vi "CU_Main_Function.vi"(8 "Stop Button Ref":refnum<vi>, 10 "Indicator Refs in":T4, 11 "Classifier Metaparameters in":T1={"Training Data Path"=path "", "Test Data Path"=path "", "True Labels Path"=path "", "SVM ClassifierOptions"={"Kernel"=enum."Linear", "Degree"=3, "Gamma"=1.0, "Coefficient"=0.0, "Sigma"=1.0, "Cache(MB)"=200.0}, "% of redundant features"=0.0, "Use equal number of trials?"=FALSE, "ClassifierQualityMeasure"=enum."Accuracy"} {"% of redundant features" min=0.0 max=100.0 step=1.0 scale=0.0..100.0}) -> (2 "Accuracies String out":string[](array[string]), 3 "Accuracies out":dbl[](array[numeric]) caption="Точность" format="%#_3g")   [LabVIEW 2016, in "Classifier.lvlib"]
uses:
  CU_metaIndicators.ctl
  CU_metaParameters.ctl
  <vilib>/vision/Classification.llb/IMAQ SVM Kernel Options.ctl
  CU_ClassifierQualityMeasure.ctl
  CU_ApplicationState.ctl
  ClassifierClass.lvclass
  ClassifierClass.lvclass/ClassifierClass.ctl
  CU_DataTypes.ctl
  CU_ClassifierTypes.ctl
  Classifier.lvlib
panel:
  out "Num of trials of each class":i32[](array[numeric]) caption="Число проб каждого класса"
  out "Num of Classes":i32 caption="Число классов"
  out "Number of Training Trials":i32 caption="Число обучающих проб"
  out "Number of Test Trials":i32 caption="Число тестовых проб"
  out "Number of Labels":i32 caption="Число меток классов"
  out "Iteration":i32 caption="Раунд кросс-проверки"
  out "Indices":i8[](array[numeric])
  # "This VI is a part of BCI Design library, http://www.ru-bci.org \nCopyright © 2020, Sotnikov Peter, All rights reserved. License: GNU GPLv3"
  # "Метод опорных векторов"
  # "Метод k ближайших соседей"
  # "Многослойный персептрон"
  # "Результаты чтения данных"
  # "Комитет классификаторов на основе метода опорных векторов"
  # "Классификатор на основе расстояния Махалонобиса"
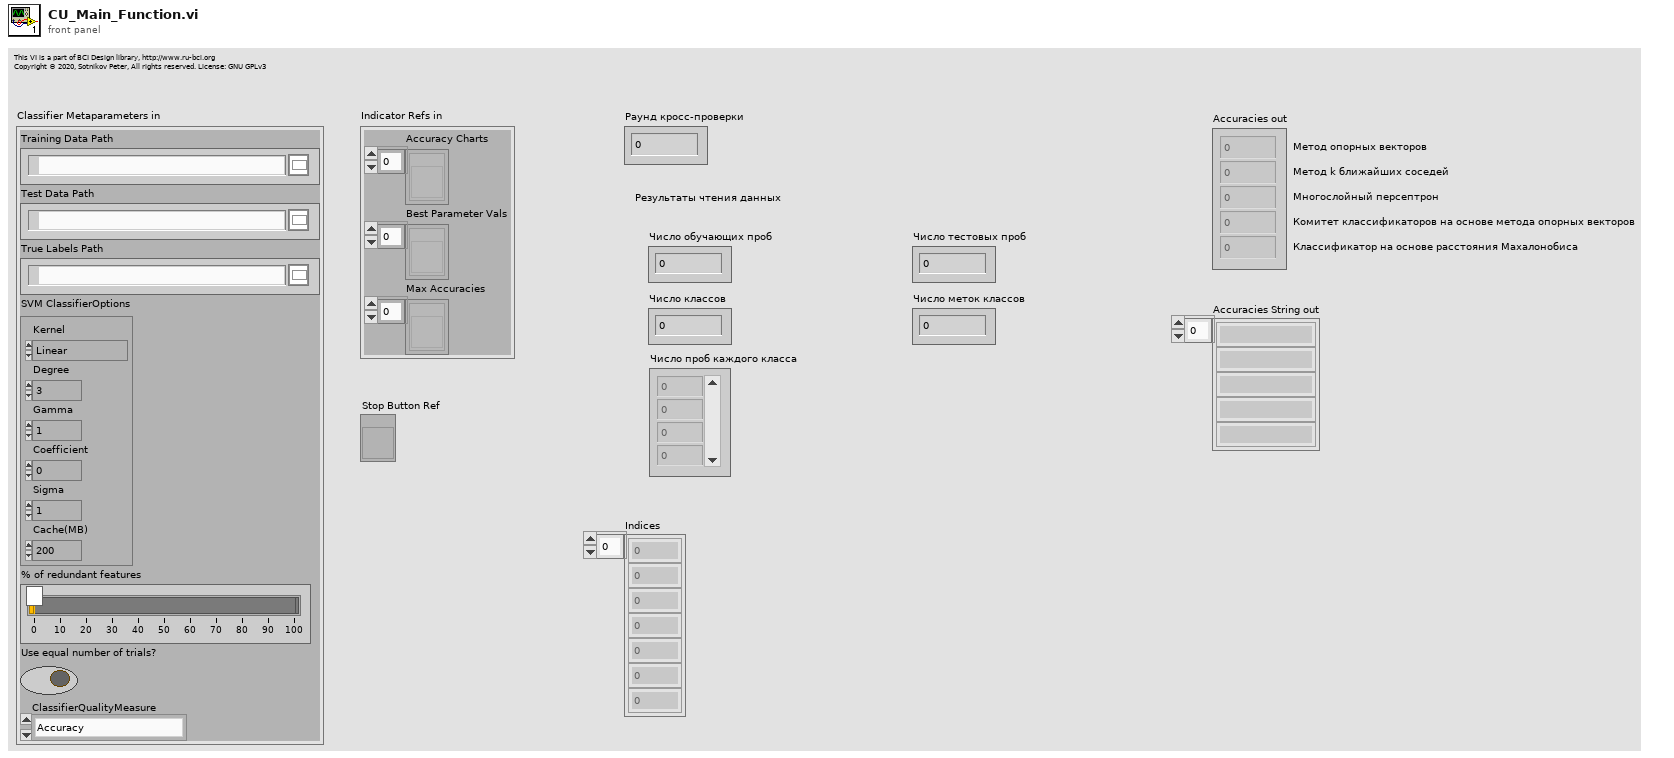
[diagram p1: front panel]
types:
  T1 = typedef "Classifier.lvlib/CU_metaParameters.ctl" = cluster{"Training Data Path":path, "Test Data Path":path, "True Labels Path":path, "SVM ClassifierOptions":T2, "% of redundant features":dbl, "Use equal number of trials?":bool, "ClassifierQualityMeasure":T3}
  T2 = typedef "IMAQ SVM Kernel Options.ctl" = cluster{"Kernel":enum32{"Linear", "Polynomial", "Gaussian", "RBF"}, "Degree":i32, "Gamma":dbl, "Coefficient":dbl, "Sigma":dbl, "Cache(MB)":dbl}
  T3 = typedef "Classifier.lvlib/CU_ClassifierQualityMeasure.ctl" = enum16{"Accuracy", "Cohen's kappa"}
  T4 = typedef "Classifier.lvlib/CU_metaIndicators.ctl" = cluster{"Accuracy Charts":refnum<vi>[], "Best Parameter Vals":refnum<vi>[], "Max Accuracies":refnum<vi>[]}
  T5 = typedef "Classifier.lvlib/CU_ApplicationState.ctl" = enum16{"Initialiaze", "Work", "On test data", "Stop", "InitCrossValidation", "CrossValidation"}
  T6 = typedef "Classifier.lvlib/CU_DataTypes.ctl" = enum16{"Training Data", "Test Data", "Training Data (cross-check)", "Test Data (cross-check)"}
  T7 = typedef "Classifier.lvlib/CU_ClassifierTypes.ctl" = enum16{"Multilayer perceptron", "k NN Classifier", "SVM Committee", "Mahalanobis distance", "SVM Classifier"}
  T8 = cluster{"Training Data Path":path, "Test Data Path":path, "True Labels Path":path}
  T9 = cluster{"Number of Classes":i32, "NumberOfTrials":i32, "NumberOfTrials":i32, "Number of labels":i32}
  T10 = typedef "IMAQ Classifier Session.ctl" = refnum<k1>
  T11 = typedef "NILabs_MLT.lvlib/ml_BP_Project.ctl" = cluster{"Training Data":T12, "Normalize Info":T13, "3-layer NN":T14, "Ternimal Condition":T15}
  T12 = typedef "NILabs_MLT.lvlib/ml_BP_Data.ctl" = cluster{"dim in":i32, "dim out":i32, "# samples":i32, "Input":dbl[][], "Output":dbl[][]}
  T13 = typedef "NILabs_MLT.lvlib/ml_BP_Normalize Data.ctl" = cluster{"input min":dbl[], "input max":dbl[], "output min":dbl[], "output max":dbl[]}
  T14 = typedef "NILabs_MLT.lvlib/ml_BP_3layer Feedforward.ctl" = cluster{"# input neuron ":i32, "# hidden neuron":i32, "# output neuron":i32, "Weight (I->H)":dbl[][], "Weight (H->O)":dbl[][], "Output":dbl[][], "Hidden Out":dbl[][], "Derivation Output":dbl[][], "Derivation Hidden":dbl[][], "dw (I->H)":dbl[][], "dw (H->O)":dbl[][]}
  T15 = typedef "NILabs_MLT.lvlib/ml_BP_Terminal Condition.ctl" = cluster{"min MSE":dbl, "min delta MSE":dbl, "min step length":dbl, "max iteration":dbl}
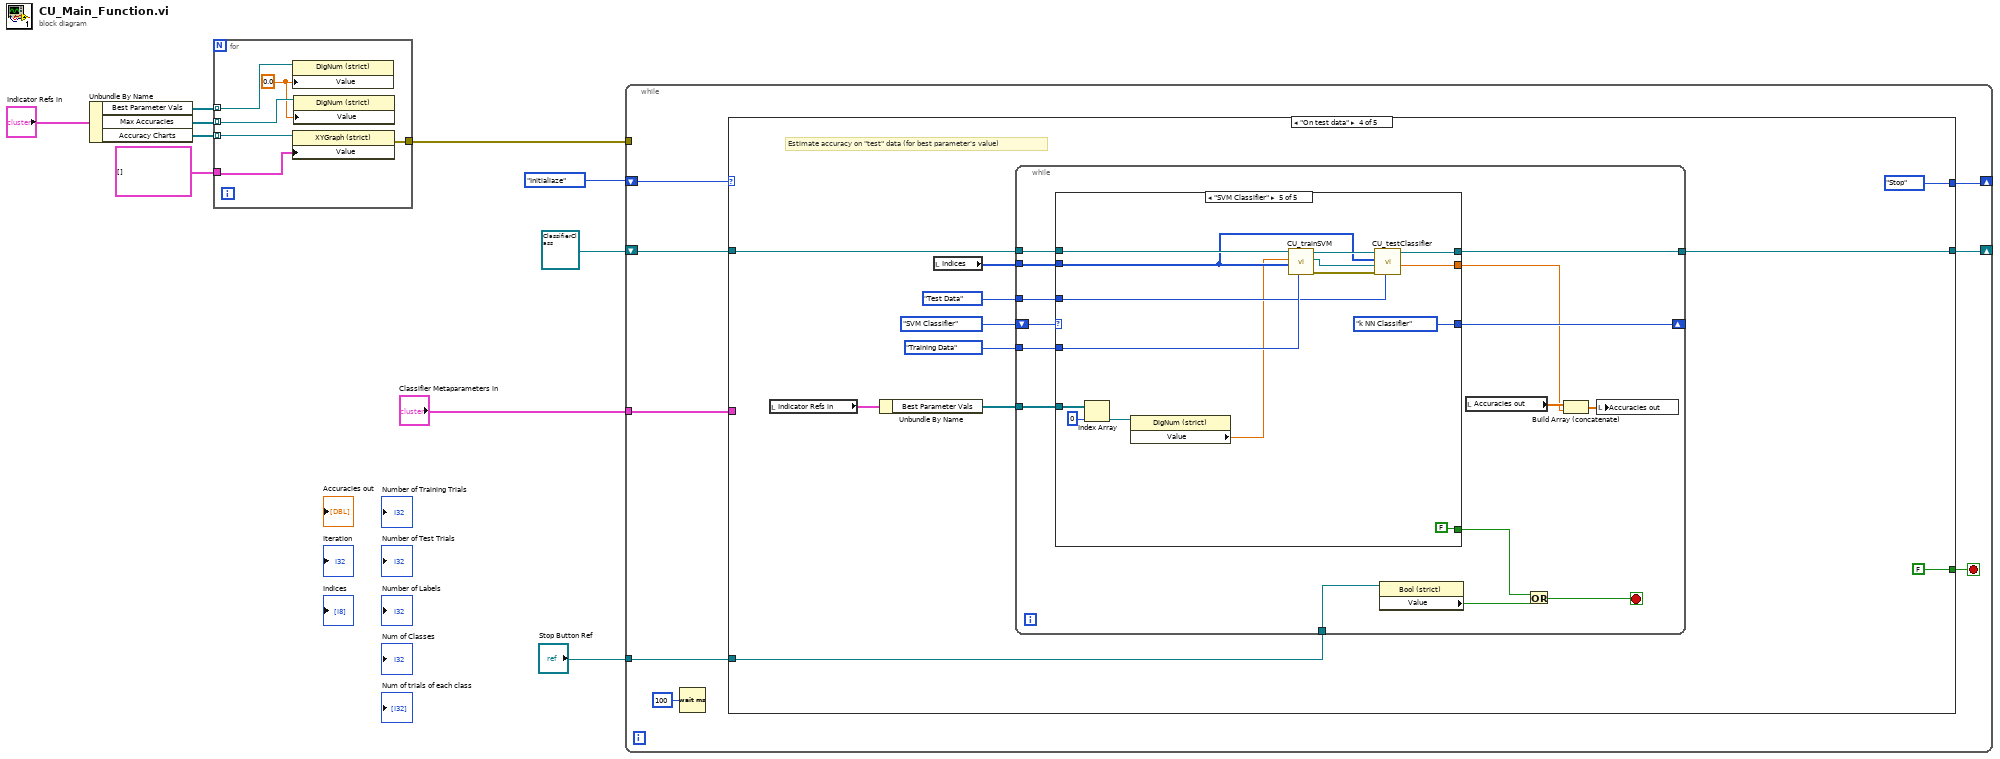
[diagram p0: block diagram]
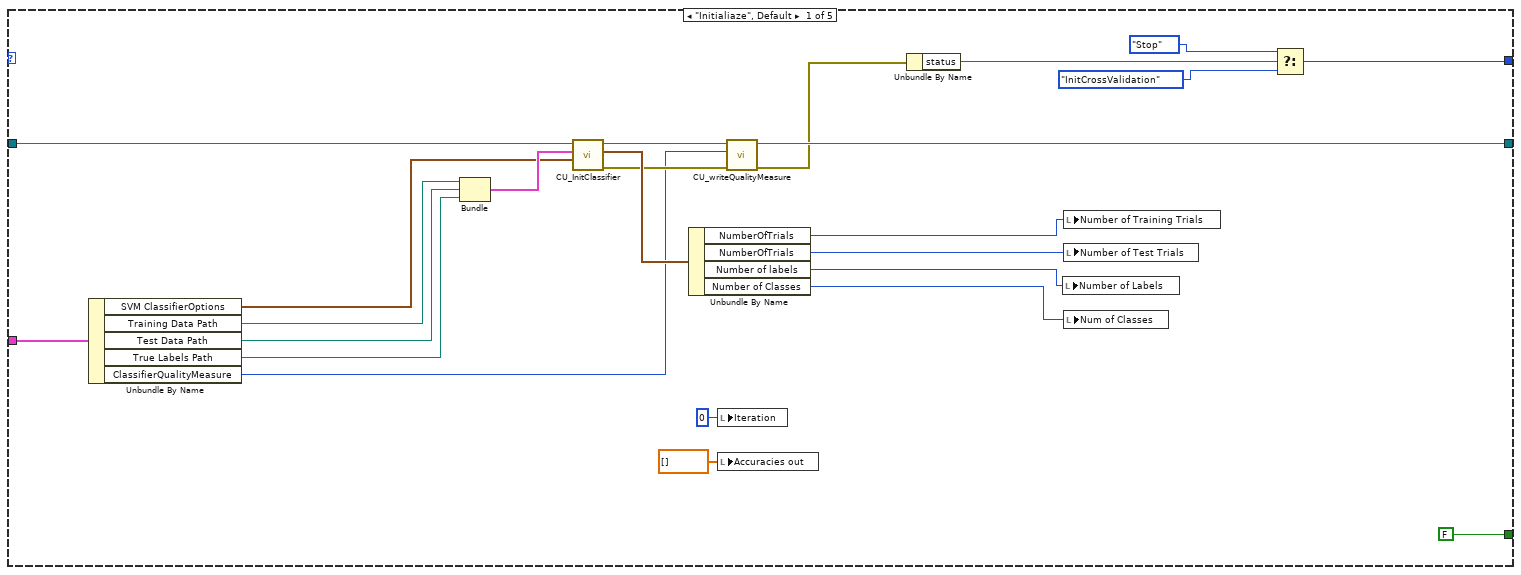
[diagram p2: hidden frame]
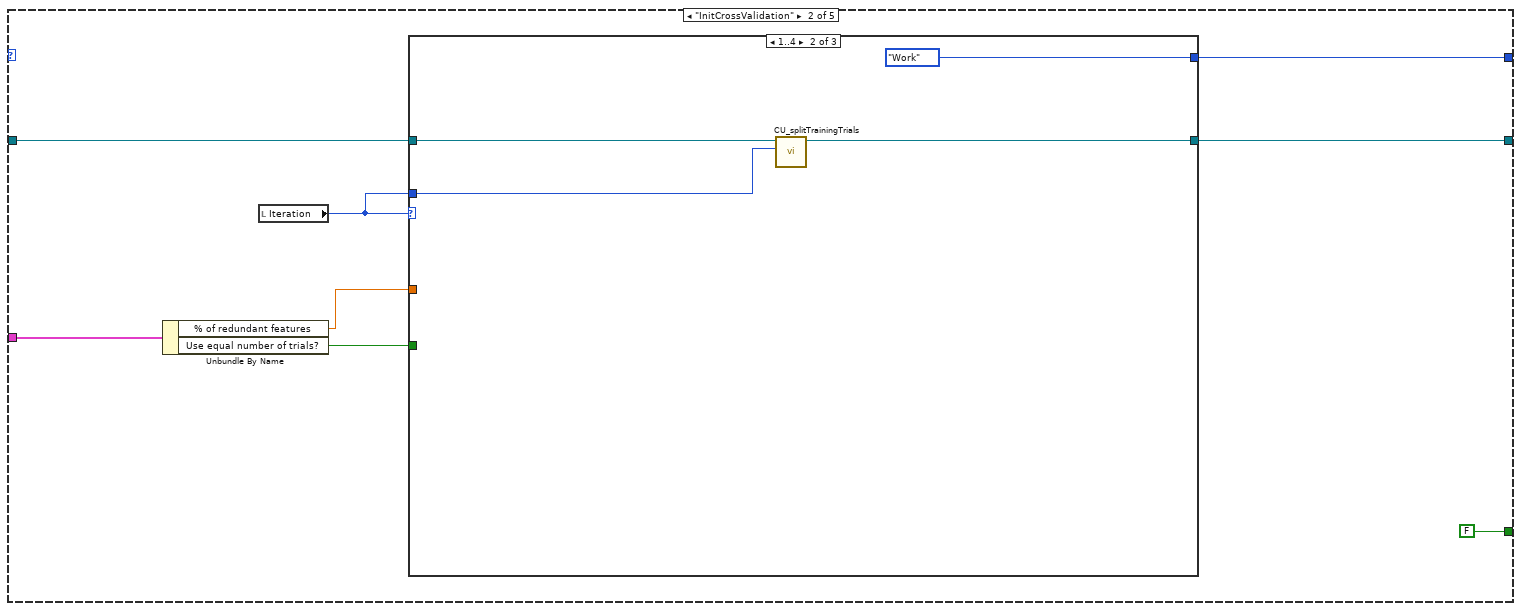
[diagram p3: hidden frame]
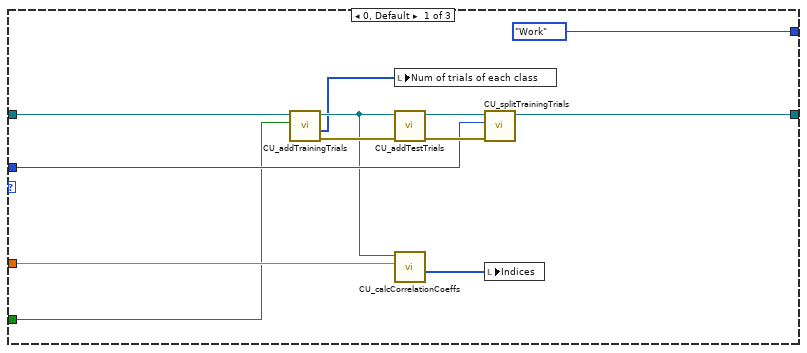
[diagram p4: hidden frame]
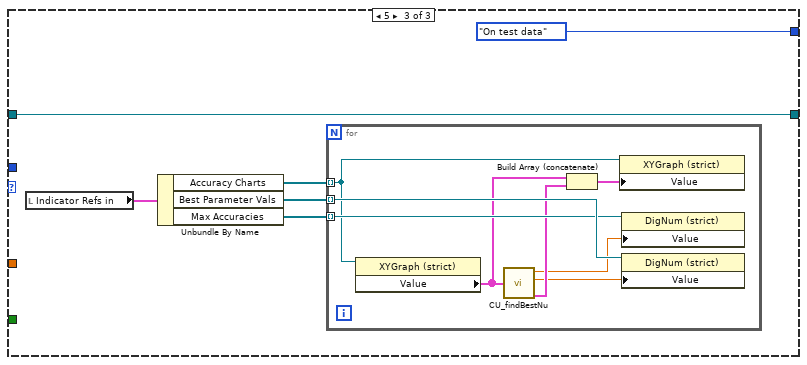
[diagram p5: hidden frame]
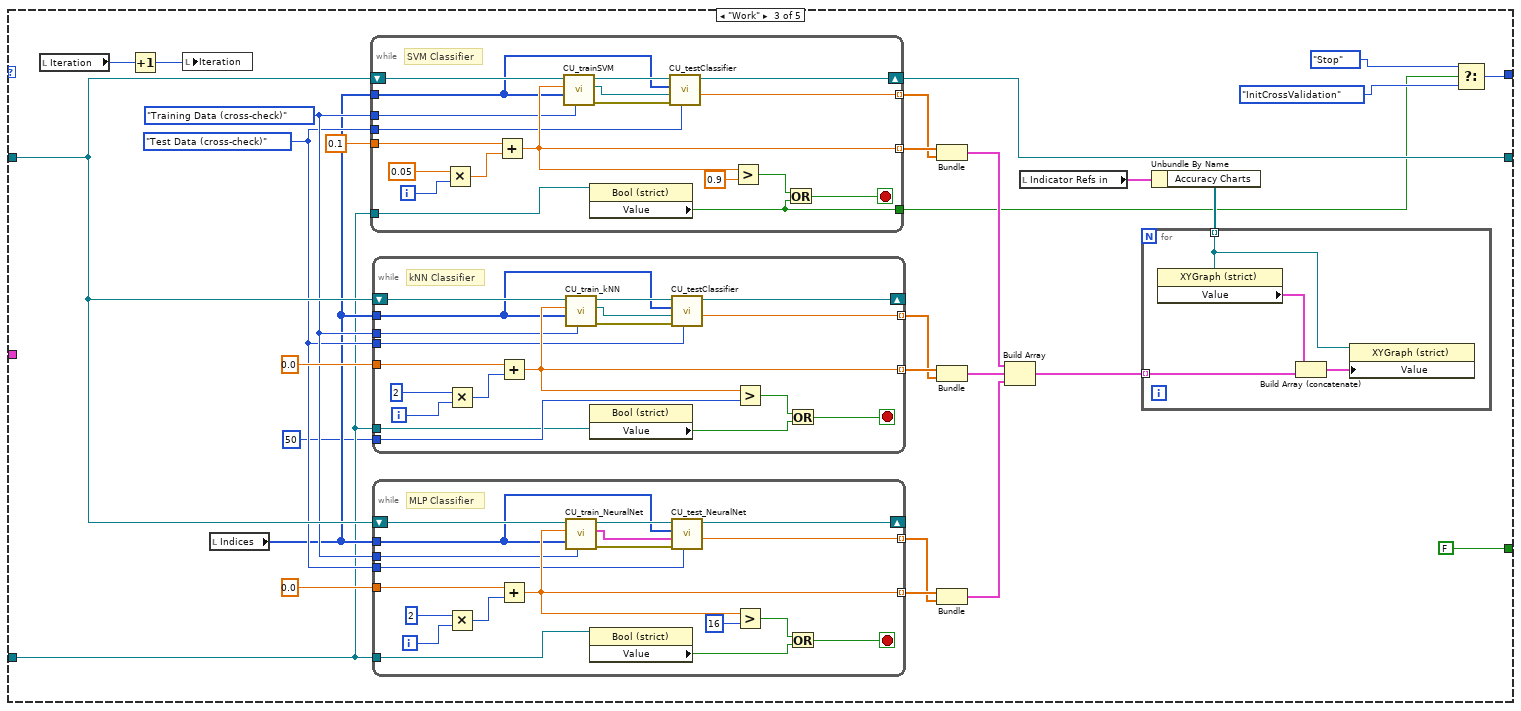
[diagram p6: hidden frame]
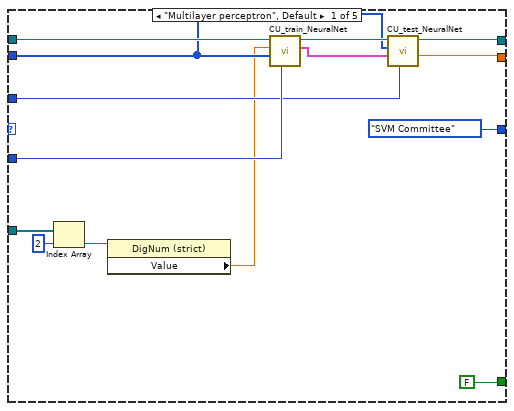
[diagram p7: hidden frame]
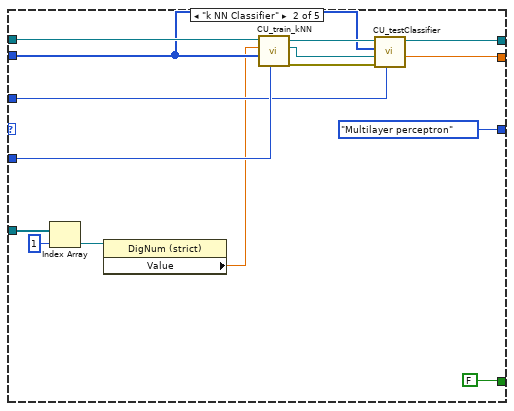
[diagram p8: hidden frame]
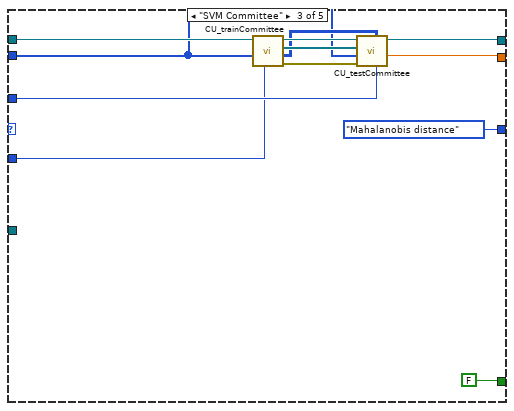
[diagram p9: hidden frame]
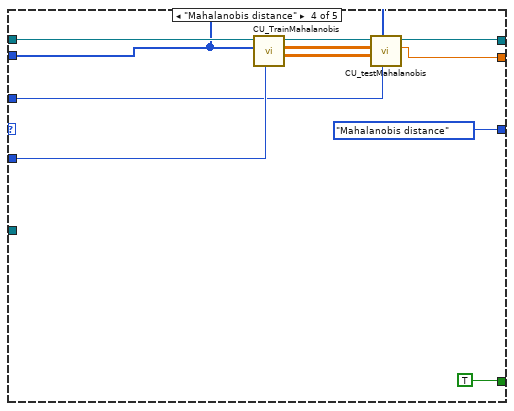
[diagram p10: hidden frame]
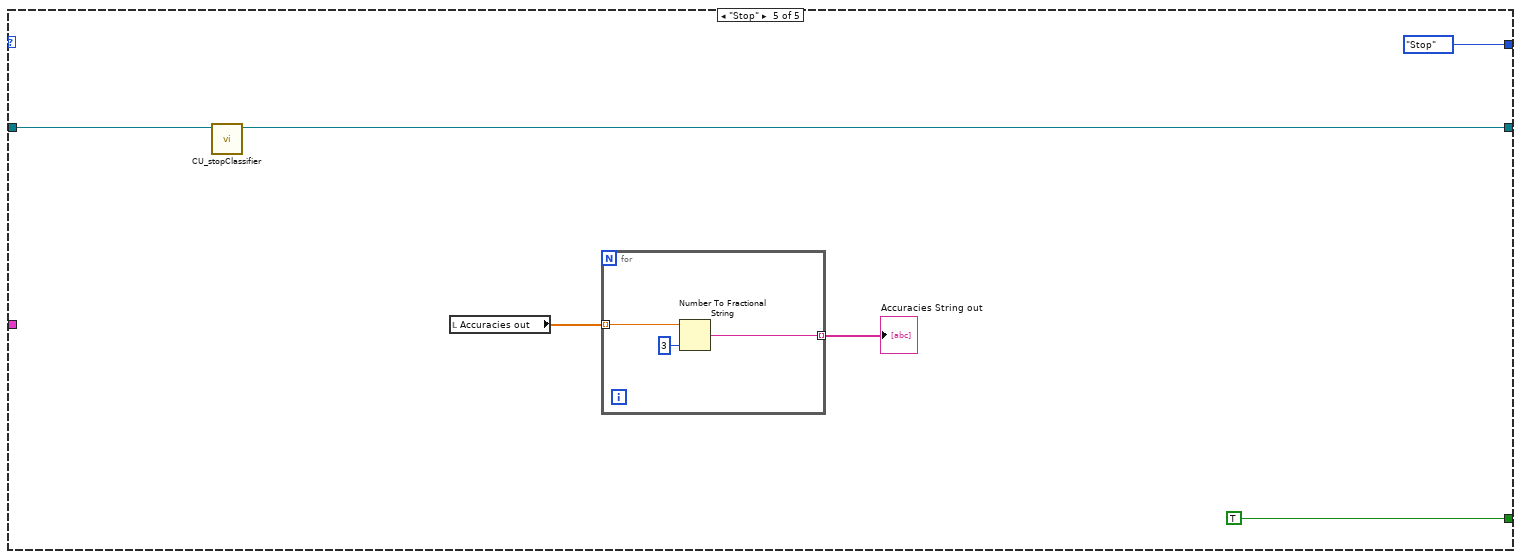
[diagram p11: hidden frame]
diagram:
  n1 = Unbundle By Name("Indicator Refs in") -> ("Best Parameter Vals"=w4:refnum<vi>[], "Max Accuracies"=w3:refnum<vi>[], "Accuracy Charts"=w7:refnum<vi>[])
  n2 = for {
    tunnel: w7 -> [w16] mode=indexing
    tunnel: [w15] -> w6
    tunnel: w4 -> [w14] mode=indexing
    tunnel: w3 -> [w13] mode=indexing
    tunnel: cluster{dbl[], dbl[]}[] [] ("Value") -> [w11]
    w12 = 0.0 ("Value")
    n3 = property class="XYGraph (strict)"(reference=w16, "Value"=w11) -> (error out=w15:errorcluster)  [unwired: 1 in, 1 out]
    n4 = property class="DigNum (strict)"(reference=w14, "Value"=w12) -> ()  [unwired: 1 in, 2 out]
    n5 = property class="DigNum (strict)"(reference=w13, "Value"=w12) -> ()  [unwired: 1 in, 2 out]
  }
  n6 = while {
    shift-right: [w23] -> _
    shift-left: CU_ApplicationState."Initialiaze" ("Application State") -> [w24]
    shift-right: [w19] -> _
    shift-left: refnum<class "ClassifierClass.lvclass"> refnum ("ClassifierClass.lvclass") -> [w20]
    tunnel: w6 -> [_]
    tunnel: "Stop Button Ref" -> [w18]
    tunnel: "Classifier Metaparameters in" -> [w17]
    stop <- w22 stop-if-true
    n7 = Wait (ms)(milliseconds to wait=u32 100) -> ()  [unwired: 1 out]
    n8 = case shown="\"On test data\"" w24 {
      tunnel: [w48 w55 w89 CU_ApplicationState."Stop" ("f") CU_ApplicationState."Stop" ("f")] -> w23
      tunnel: [FALSE FALSE FALSE FALSE TRUE] -> w22
      tunnel: w20 -> [w46 w56 w107 w183 w273]
      tunnel: [w26 w53 w113 w184 w272] -> w19
      tunnel: w18 -> [_ _ w92 w177 _]
      tunnel: w17 -> [w36 w51 _ _ _]
      frame "Initialiaze", Default {
        n9 = Unbundle By Name(w36) -> ("SVM ClassifierOptions"=w32:T2, "Training Data Path"=w35:path, "Test Data Path"=w34:path, "True Labels Path"=w33:path, "ClassifierQualityMeasure"=w27:T3)
        n10 = Bundle("Training Data Path"=w35, "Test Data Path"=w34, "True Labels Path"=w33) -> (w43:T8)  [unwired: 1 in]
        n11 = call "CU_InitClassifier.vi"("Kernel Options"=w32, "Paths"=w43, "ClassifierClass in"=w46) -> ("error out"=w28:errorcluster, "Number of Trials"=w41:T9, "ClassifierClass out"=w29:refnum<class "ClassifierClass.lvclass">)  [unwired: 6 in]
        n12 = Unbundle By Name(w41) -> ("NumberOfTrials"=w40:i32, "NumberOfTrials"=w39:i32, "Number of labels"=w38:i32, "Number of Classes"=w37:i32)
        n13 = local write "Iteration"(0 ("Iteration")) -> ()
        n14 = local write "Accuracies out"(dbl[] [] ("Accuracies out")) -> ()
        n15 = call "CU_writeQualityMeasure.vi"("error in (no error)"=w28, "ClassifierQualityMeasure in"=w27, "ClassifierClass in"=w29) -> ("error out"=w25:errorcluster, "ClassifierClass out"=w26:refnum<class "ClassifierClass.lvclass">)  [unwired: 7 in]
        n16 = Unbundle By Name(w25) -> ("status"=w42:bool)
        n17 = local write "Number of Labels"(w38) -> ()
        n18 = local write "Number of Training Trials"(w40) -> ()
        n19 = local write "Number of Test Trials"(w39) -> ()
        n20 = local write "Num of Classes"(w37) -> ()
        n21 = Select(t=CU_ApplicationState."Stop" ("Application State"), s=w42, f=CU_ApplicationState."InitCrossValidation") -> (s? t:f=w48:T5)
      }
      frame "InitCrossValidation" {
        n22 = Unbundle By Name(w51) -> ("% of redundant features"=w50:dbl, "Use equal number of trials?"=w49:bool)
        n23 = local read "Iteration"() -> (w52:i32)
        n24 = case shown="1..4" w52 {
          tunnel: w56 -> [w68 w72 w78]
          tunnel: [w65 w71 w78] -> w53
          tunnel: w52 -> [w63 w70 _]
          tunnel: [CU_ApplicationState."Work" ("Application State") CU_ApplicationState."Work" ("Application State") CU_ApplicationState."On test data" ("Application State")] -> w55
          tunnel: w50 -> [w59 _ _]
          tunnel: w49 -> [w58 _ _]
          frame 0, Default {
            n25 = call "CU_addTrainingTrials.vi"("Use equal number of trials?"=w58, "ClassifierClass in"=w68) -> ("error out"=w67:errorcluster, "Num of Trials of each Class"=w57:i32[], "ClassifierClass out"=w61:refnum<class "ClassifierClass.lvclass">)  [unwired: 6 in, 1 out]
            n26 = local write "Num of trials of each class"(w57) -> ()
            n27 = call "CU_addTestTrials.vi"("error in (no error)"=w67, "ClassifierClass in"=w61) -> ("error out"=w64:errorcluster, "ClassifierClass out"=w66:refnum<class "ClassifierClass.lvclass">)  [unwired: 6 in, 2 out]
            n28 = call "CU_calcCorrelationCoeffs.vi"("Percent in"=w59, "ClassifierClass in"=w61) -> ("Indicies"=w60:i16[])  [unwired: 6 in, 3 out]
            n29 = call "CU_splitTrainingTrials.vi"("error in (no error)"=w64, "Iteration"=w63, "ClassifierClass in"=w66) -> ("ClassifierClass out"=w65:refnum<class "ClassifierClass.lvclass">)  [unwired: 5 in, 3 out]
            n30 = local write "Indices"(w60) -> ()
          }
          frame 1..4 {
            n31 = call "CU_splitTrainingTrials.vi"("Iteration"=w70, "ClassifierClass in"=w72) -> ("ClassifierClass out"=w71:refnum<class "ClassifierClass.lvclass">)  [unwired: 6 in, 3 out]
          }
          frame 5 {
            n32 = local read "Indicator Refs in"() -> (w76:T4)
            n33 = Unbundle By Name(w76) -> ("Accuracy Charts"=w75:refnum<vi>[], "Best Parameter Vals"=w74:refnum<vi>[], "Max Accuracies"=w73:refnum<vi>[])
            n34 = for {
              tunnel: w75 -> [w84] mode=indexing
              tunnel: w74 -> [w86] mode=indexing
              tunnel: w73 -> [w85] mode=indexing
              n35 = property class="XYGraph (strict)"(reference=w84) -> ("Value"=w82:cluster{dbl[], dbl[]}[])  [unwired: 1 in, 2 out]
              n36 = call "CU_findBestNu.vi"("Accuracy Graph"=w82) -> ("Max Average Accuracy"=w80:dbl, "Best Value"=w79:dbl, "Average Accuracy"=w83:cluster{dbl[], dbl[]})  [unwired: 7 in]
              n37 = Build Array (concatenate)(w82, w83) -> (w81:cluster{dbl[], dbl[]}[])
              n38 = property class="XYGraph (strict)"(reference=w84, "Value"=w81) -> ()  [unwired: 1 in, 2 out]
              n39 = property class="DigNum (strict)"(reference=w85, "Value"=w80) -> ()  [unwired: 1 in, 2 out]
              n40 = property class="DigNum (strict)"(reference=w86, "Value"=w79) -> ()  [unwired: 1 in, 2 out]
            }
          }
        }
      }
      frame "Work" {
        w101 = CU_DataTypes."Test Data (cross-check)" ("DataTypes")
        w102 = CU_DataTypes."Training Data (cross-check)" ("DataTypes")
        n41 = local read "Iteration"() -> (w110:i32)
        n42 = Increment(x=w110) -> (x+1=w109:i32)
        n43 = local write "Iteration"(w109) -> ()
        n44 = local read "Indices"() -> (w100:i8[])
        n45 = while {
          tunnel: 0.1 -> [w172]
          tunnel: [w170] -> w111 mode=indexing
          shift-right: [w169] -> w113
          shift-left: w107 -> [w176]
          tunnel: [w163] -> w112 mode=indexing
          tunnel: w102 -> [w162]
          tunnel: w101 -> [w161]
          tunnel: w100 -> [w160]
          tunnel: w92 -> [w159]
          tunnel: [w158] -> w88
          i -> [w175]
          stop <- w166 stop-if-true
          # "SVM Classifier"
          n46 = Multiply(x=0.05, y=w175) -> (x*y=w173:dbl)
          n47 = Add(x=w172, y=w173) -> (x+y=w163:dbl)
          n48 = call "CU_trainSVM.vi"("Train Data"=w162, "Indices"=w160, "Nu Value"=w163, "ClassifierClass in"=w176) -> ("error out"=w165:errorcluster, "Classifier Session out"=w164:T10, "ClassifierClass out"=w171:refnum<class "ClassifierClass.lvclass">)  [unwired: 5 in]
          n49 = property class="Bool (strict)"(reference=w159) -> ("Value"=w158:bool)  [unwired: 1 in, 2 out]
          n50 = call "CU_testClassifier.vi"("DataTypes"=w161, "error in"=w165, "Classifier Session Ref"=w164, "Indices"=w160, "ClassifierClass in"=w171) -> ("Accuracy"=w170:dbl, "ClassifierClass out"=w169:refnum<class "ClassifierClass.lvclass">)  [unwired: 3 in, 2 out]
          n51 = Greater?(x=w163, y=0.9) -> (0:w167:bool)
          n52 = Or(x=w167, y=w158) -> (x .or. y?=w166:bool)
        }
        n53 = while {
          tunnel: 0.0 -> [w153]
          tunnel: [w151] -> w105 mode=indexing
          shift-right: [w150] -> _
          shift-left: w107 -> [w157]
          tunnel: 50 -> [w145]
          tunnel: [w144] -> w106 mode=indexing
          tunnel: w102 -> [w143]
          tunnel: w101 -> [w142]
          tunnel: w100 -> [w141]
          tunnel: w92 -> [w139]
          i -> [w156]
          stop <- w148 stop-if-true
          # "kNN Classifier"
          n54 = Multiply(x=2, y=w156) -> (x*y=w154:i32)
          n55 = Add(x=w153, y=w154) -> (x+y=w144:dbl)
          n56 = call "CU_train_kNN.vi"("DataTypes"=w143, "Indices"=w141, "k value"=w144, "ClassifierClass in"=w157) -> ("error out"=w147:errorcluster, "Classifier Session out"=w146:T10, "ClassifierClass out"=w152:refnum<class "ClassifierClass.lvclass">)  [unwired: 5 in]
          n57 = property class="Bool (strict)"(reference=w139) -> ("Value"=w140:bool)  [unwired: 1 in, 2 out]
          n58 = call "CU_testClassifier.vi"("DataTypes"=w142, "error in"=w147, "Classifier Session Ref"=w146, "Indices"=w141, "ClassifierClass in"=w152) -> ("Accuracy"=w151:dbl, "ClassifierClass out"=w150:refnum<class "ClassifierClass.lvclass">)  [unwired: 3 in, 2 out]
          n59 = Greater?(x=w144, y=w145) -> (0:w149:bool)
          n60 = Or(x=w149, y=w140) -> (x .or. y?=w148:bool)
        }
        n61 = while {
          tunnel: [w134] -> w93 mode=indexing
          shift-right: [w133] -> _
          shift-left: w107 -> [w138]
          tunnel: [w128] -> w103 mode=indexing
          tunnel: 0.0 -> [w127]
          tunnel: w102 -> [w124]
          tunnel: w101 -> [w123]
          tunnel: w100 -> [w122]
          tunnel: w92 -> [w121]
          i -> [w137]
          stop <- w131 stop-if-true
          # "MLP Classifier"
          n62 = Multiply(x=2, y=w137) -> (x*y=w136:i32)
          n63 = Add(x=w127, y=w136) -> (x+y=w128:dbl)
          n64 = call "CU_train_NeuralNet.vi"("DataTypes"=w124, "Indices"=w122, "# of hidden neuron"=w128, "ClassifierClass in"=w138) -> ("error out"=w130:errorcluster, "ANN out"=w129:T11, "ClassifierClass out"=w135:refnum<class "ClassifierClass.lvclass">)  [unwired: 4 in, 1 out]
          n65 = property class="Bool (strict)"(reference=w121) -> ("Value"=w120:bool)  [unwired: 1 in, 2 out]
          n66 = call "CU_test_NeuralNet.vi"("DataTypes"=w123, "error in"=w130, "ANN in"=w129, "Indices"=w122, "ClassifierClass in"=w135) -> ("Accuracy"=w134:dbl, "ClassifierClass out"=w133:refnum<class "ClassifierClass.lvclass">)  [unwired: 3 in, 2 out]
          n67 = Greater?(x=w128, y=16) -> (0:w132:bool)
          n68 = Or(x=w132, y=w120) -> (x .or. y?=w131:bool)
        }
        n69 = Bundle(w112, w111) -> (w97:cluster{dbl[], dbl[]})  [unwired: 1 in]
        n70 = Bundle(w106, w105) -> (w98:cluster{dbl[], dbl[]})  [unwired: 1 in]
        n71 = Bundle(w103, w93) -> (w96:cluster{dbl[], dbl[]})  [unwired: 1 in]
        n72 = Build Array(w97, w98, w96) -> (w94:cluster{dbl[], dbl[]}[])
        n73 = local read "Indicator Refs in"() -> (w99:T4)
        n74 = Unbundle By Name(w99) -> ("Accuracy Charts"=w95:refnum<vi>[])
        n75 = for {
          tunnel: w95 -> [w119] mode=indexing
          tunnel: w94 -> [w117] mode=indexing
          n76 = property class="XYGraph (strict)"(reference=w119) -> ("Value"=w118:cluster{dbl[], dbl[]}[])  [unwired: 1 in, 2 out]
          n77 = Build Array (concatenate)(w118, w117) -> (w116:cluster{dbl[], dbl[]}[])
          n78 = property class="XYGraph (strict)"(reference=w119, "Value"=w116) -> ()  [unwired: 1 in, 2 out]
        }
        n79 = Select(t=CU_ApplicationState."Stop" ("Application State"), s=w88, f=CU_ApplicationState."InitCrossValidation") -> (s? t:f=w89:T5)
      }
      frame "On test data" {
        # "Estimate accuracy on \"test\" data (for best parameter's value)"
        n80 = local read "Indicator Refs in"() -> (w179:T4)
        n81 = Unbundle By Name(w179) -> ("Best Parameter Vals"=w178:refnum<vi>[])
        n82 = local read "Indices"() -> (w180:i8[])
        n83 = while {
          shift-right: [w201] -> _
          shift-left: CU_ClassifierTypes."SVM Classifier" ("ClassifierTypes") -> [w202]
          tunnel: w183 -> [w200]
          tunnel: [w199] -> w184
          tunnel: CU_DataTypes."Training Data" ("Train Data") -> [w198]
          tunnel: CU_DataTypes."Test Data" ("DataTypes") -> [w197]
          tunnel: w180 -> [w193]
          tunnel: w178 -> [w192]
          tunnel: w177 -> [w191]
          stop <- w188 stop-if-true
          n84 = case shown="\"SVM Classifier\"" w202 {
            tunnel: [FALSE FALSE FALSE TRUE FALSE] -> w189
            tunnel: [CU_ClassifierTypes."SVM Committee" ("ClassifierTypes") CU_ClassifierTypes."Multilayer perceptron" ("ClassifierTypes") CU_ClassifierTypes."Mahalanobis distance" ("ClassifierTypes") CU_ClassifierTypes."Mahalanobis distance" ("ClassifierTypes") CU_ClassifierTypes."k NN Classifier" ("ClassifierTypes")] -> w201
            tunnel: w200 -> [w214 w225 w238 w251 w266]
            tunnel: [w212 w226 w237 w250 w265] -> w199
            tunnel: w198 -> [w209 w223 w234 w247 w263]
            tunnel: w197 -> [w208 w222 w235 w246 w262]
            tunnel: [w210 w224 w233 w245 w261] -> w194
            tunnel: w193 -> [w207 w221 w232 w244 w260]
            tunnel: w192 -> [w206 w220 _ _ w258]
            frame "Multilayer perceptron", Default {
              n85 = Index Array(array=w206, index=2) -> (element=w204:refnum<vi>)
              n86 = property class="DigNum (strict)"(reference=w204) -> ("Value"=w203:dbl)  [unwired: 1 in, 2 out]
              n87 = call "CU_train_NeuralNet.vi"("DataTypes"=w209, "Indices"=w207, "# of hidden neuron"=w203, "ClassifierClass in"=w214) -> ("ANN out"=w211:T11, "ClassifierClass out"=w213:refnum<class "ClassifierClass.lvclass">)  [unwired: 4 in, 2 out]
              n88 = call "CU_test_NeuralNet.vi"("DataTypes"=w208, "ANN in"=w211, "Indices"=w207, "ClassifierClass in"=w213) -> ("Accuracy"=w210:dbl, "ClassifierClass out"=w212:refnum<class "ClassifierClass.lvclass">)  [unwired: 4 in, 2 out]
            }
            frame "k NN Classifier" {
              n89 = Index Array(array=w220, index=1) -> (element=w218:refnum<vi>)
              n90 = property class="DigNum (strict)"(reference=w218) -> ("Value"=w217:dbl)  [unwired: 1 in, 2 out]
              n91 = call "CU_train_kNN.vi"("DataTypes"=w223, "Indices"=w221, "k value"=w217, "ClassifierClass in"=w225) -> ("error out"=w228:errorcluster, "Classifier Session out"=w229:T10, "ClassifierClass out"=w227:refnum<class "ClassifierClass.lvclass">)  [unwired: 5 in]
              n92 = call "CU_testClassifier.vi"("DataTypes"=w222, "error in"=w228, "Classifier Session Ref"=w229, "Indices"=w221, "ClassifierClass in"=w227) -> ("Accuracy"=w224:dbl, "ClassifierClass out"=w226:refnum<class "ClassifierClass.lvclass">)  [unwired: 3 in, 2 out]
            }
            frame "SVM Committee" {
              n93 = call "CU_trainCommittee.vi"("DataTypes"=w234, "Indices"=w232, "ClassifierClass in"=w238) -> ("error out"=w240:errorcluster, "Classification Distribution"=w236:i32[][][], "Classifier Refs out"=w241:T10[], "ClassifierClass out"=w239:refnum<class "ClassifierClass.lvclass">)  [unwired: 5 in]
              n94 = call "CU_testCommittee.vi"("ClassifierClass in"=w239, "Classifier Refs in"=w241, "Indices"=w232, "error in"=w240, "Classification Distribution"=w236, "DataTypes"=w235) -> ("ClassifierClass out"=w237:refnum<class "ClassifierClass.lvclass">, "Accuracy"=w233:dbl)  [unwired: 2 out]
            }
            frame "Mahalanobis distance" {
              n95 = call "CU_TrainMahalanobis.vi"("DataTypes"=w247, "Indices"=w244, "ClassifierClass in"=w251) -> ("Mean vectors"=w252:dbl[][], "Covariance matricies"=w253:dbl[][][], "ClassifierClass out"=w254:refnum<class "ClassifierClass.lvclass">)  [unwired: 5 in, 1 out]
              n96 = call "CU_testMahalanobis.vi"("DataTypes"=w246, "Indices"=w244, "Mean vectors"=w252, "Covariance matricies"=w253, "ClassifierClass in"=w254) -> ("Accuracy"=w245:dbl, "ClassifierClass out"=w250:refnum<class "ClassifierClass.lvclass">)  [unwired: 3 in, 2 out]
            }
            frame "SVM Classifier" {
              n97 = Index Array(array=w258, index=0) -> (element=w256:refnum<vi>)
              n98 = property class="DigNum (strict)"(reference=w256) -> ("Value"=w255:dbl)  [unwired: 1 in, 2 out]
              n99 = call "CU_trainSVM.vi"("Train Data"=w263, "Indices"=w260, "Nu Value"=w255, "ClassifierClass in"=w266) -> ("error out"=w268:errorcluster, "Classifier Session out"=w269:T10, "ClassifierClass out"=w267:refnum<class "ClassifierClass.lvclass">)  [unwired: 5 in]
              n100 = call "CU_testClassifier.vi"("DataTypes"=w262, "error in"=w268, "Classifier Session Ref"=w269, "Indices"=w260, "ClassifierClass in"=w267) -> ("Accuracy"=w261:dbl, "ClassifierClass out"=w265:refnum<class "ClassifierClass.lvclass">)  [unwired: 3 in, 2 out]
            }
          }
          n101 = property class="Bool (strict)"(reference=w191) -> ("Value"=w190:bool)  [unwired: 1 in, 2 out]
          n102 = local read "Accuracies out"() -> (w196:dbl[])
          n103 = Or(x=w189, y=w190) -> (x .or. y?=w188:bool)
          n104 = Build Array (concatenate)(w196, w194) -> (w195:dbl[])
          n105 = local write "Accuracies out"(w195) -> ()
        }
      }
      frame "Stop" {
        n106 = call "CU_stopClassifier.vi"("ClassifierClass in"=w273) -> ("ClassifierClass out"=w272:refnum<class "ClassifierClass.lvclass">)  [unwired: 9 in, 1 out]
        n107 = local read "Accuracies out"() -> (w271:dbl[])
        n108 = for {
          tunnel: w271 -> [w278] mode=indexing
          tunnel: [w276] -> w270 mode=indexing
          n109 = Number To Fractional String(number=w278, precision (6)=i16 3) -> (F-format string=w276:string)  [unwired: 2 in]
        }
        "Accuracies String out" <- w270
      }
    }
  }
